vi "niRFUtil FTW Decimating FIR Filter (real wfm).vi"(0 "Waveform In":T1 {"y" min=0 max=127 format="%.2f"; "dx" format="%^.2e"; "x0" format="%^.2e"}, 5 "Filter":T1 {"y" min=0 max=127 format="%.2f"; "dx" format="%^.2e"; "x0" format="%^.2e"}, 7 "Decimating Factor":i32=1, 9 "Offset":i32) -> (4 "Waveform Out":T1 {"y" min=0 max=127 format="%.2f"; "dx" format="%^.2e"; "x0" format="%^.2e"})   [LabVIEW 2015, in "niRFUtil.lvlib"]
doc: "(c) Copyright 2006, National Instruments, Inc. This VI may not be duplicated, sold, or distributed without written consent from National Instruments."
uses:
  niRFUtil.lvlib
  Includes/niRFUtil INC Real Waveform.ctl
  Includes/niRFUtil INC Real Array.ctl
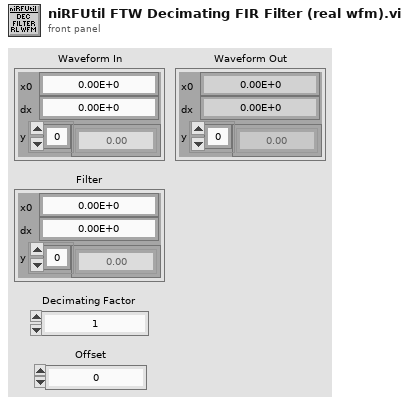
[diagram p1: front panel]
types:
  T1 = typedef "niRFUtil.lvlib/niRFUtil INC Real Waveform.ctl" = cluster{"x0":dbl, "dx":dbl, "y":T2}
  T2 = typedef "niRFUtil.lvlib/niRFUtil INC Real Array.ctl" = sgl[]
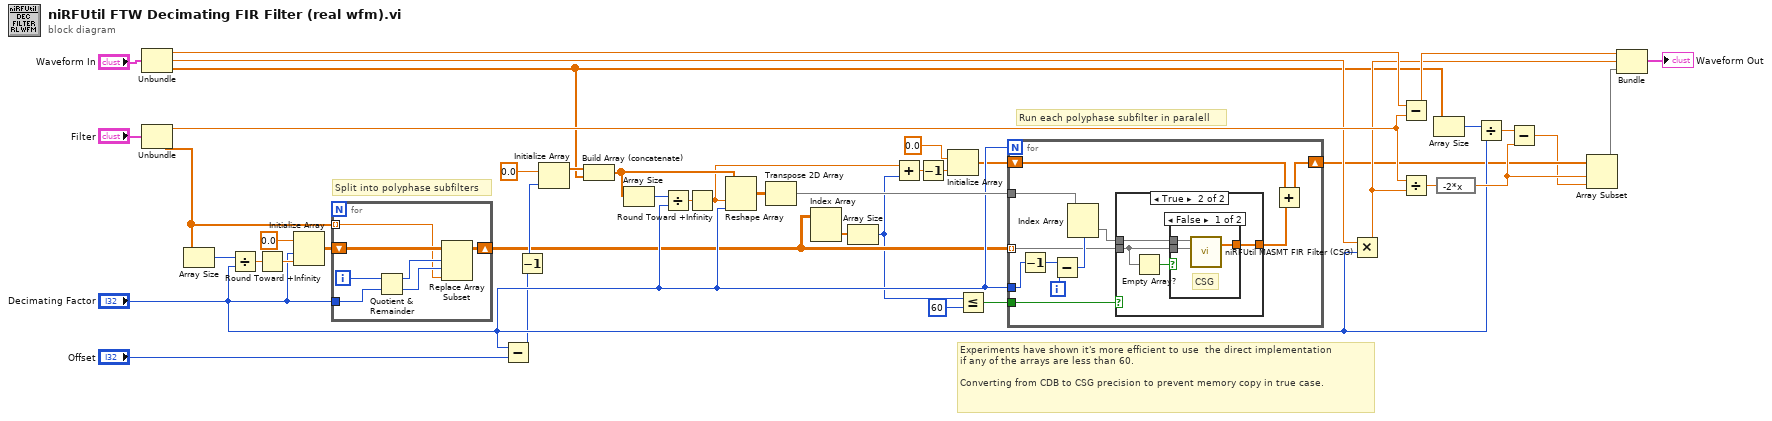
[diagram p0: block diagram]
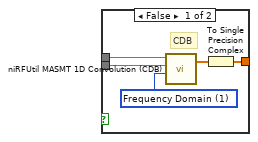
[diagram p2: hidden frame]
diagram:
  # "Experiments have shown it's more efficient to use  the direct implementation\nif any of the arrays are less than 60. \n\nConverting from CDB to CSG precision to prevent memory copy in true case."
  # "Run each polyphase subfilter in paralell"
  # "Split into polyphase subfilters"
  n1 = Unbundle("Waveform In") -> ("x0"=w33:dbl, "dx"=w27:dbl, "y"=w19:T2)
  n2 = Unbundle("Filter") -> ("x0"=w32:dbl, "y"=w38:T2)  [unwired: 1 out]
  n3 = Array Size(array=w38) -> (size(s)=w43:i32)
  n4 = Divide(x=w43, y="Decimating Factor") -> (x/y=w42:dbl)
  n5 = Round Toward +Infinity(x=w42) -> (ceil(x): smallest int >= x=w39:dbl)
  n6 = Initialize Array(sgl 0.0 ("element"), "Decimating Factor", w39) -> (w40:sgl[][])
  n7 = for {
    tunnel: w38 -> [w45] mode=indexing
    tunnel: "Decimating Factor" -> [w50]
    shift-right: [w44] -> w14
    shift-left: w40 -> [w48]
    i -> [w49]
    n8 = Quotient & Remainder(x=w49, y=w50) -> (x-y*floor(x/y)=w47:i32, floor(x/y)=w46:i32)
    n9 = Replace Array Subset(array=w48, new element=w45, index (row)=w47, index (col)=w46) -> (w44:sgl[][])
  }
  n10 = Subtract(x="Decimating Factor", y="Offset") -> (x-y=w16:i32)
  n11 = Decrement(x=w16) -> (x-1=w15:i32)
  n12 = Initialize Array(sgl 0.0 ("element"), w15) -> (w24:sgl[])
  n13 = Build Array (concatenate)(w24, w19) -> (w23:T2)
  n14 = Array Size(array=w23) -> (size(s)=w30:i32)
  n15 = Divide(x=w30, y="Decimating Factor") -> (x/y=w28:dbl)
  n16 = Round Toward +Infinity(x=w28) -> (ceil(x): smallest int >= x=w12:dbl)
  n17 = Reshape Array(w23, w12, "Decimating Factor") -> (w29:sgl[][])
  n18 = Transpose 2D Array(2D array=w29) -> (transposed array=w22:sgl[][])
  n19 = Index Array(array=w14) -> (element=w13:sgl[])  [unwired: 2 in]
  n20 = Array Size(array=w13) -> (size(s)=w2:i32)
  n21 = Add(x=w12, y=w2) -> (x+y=w11:dbl)
  n22 = Decrement(x=w11) -> (x-1=w8:dbl)
  n23 = Initialize Array(sgl 0.0, w8) -> (w10:sgl[])
  n24 = Less Or Equal?(x=w2, y=60) -> (x <= y?=w1:bool)
  n25 = for {
    N: "Decimating Factor" -> [_]
    tunnel: w14 -> [w54] mode=indexing
    tunnel: "Decimating Factor" -> [w61]
    tunnel: w22 -> [w58]
    shift-right: [w55] -> w7
    shift-left: w10 -> [w56]
    tunnel: w1 -> [w51]
    i -> [w60]
    n26 = Decrement(x=w61) -> (x-1=w59:i32)
    n27 = Subtract(x=w59, y=w60) -> (x-y=w57:i32)
    n28 = Index Array(array=w58, index (row)=w57) -> (element=w53:sgl[])  [unwired: 1 in]
    n29 = case shown="True" w51 {
      tunnel: [w62 w70] -> w52
      tunnel: w53 -> [w64 w69]
      tunnel: w54 -> [w65 w67]
      frame False {
        w66 = 1 items=["Direct", "Frequency Domain"] ("algorithm")
        # "CDB"
        n30 = call "niRFUtil MASMT 1D Convolution (CDB).vi"("algorithm"=w66, "Y"=w65, "X"=w64) -> ("X * Y"=w63:cdb[])  [unwired: 7 in, 1 out]
        n31 = To Single Precision Complex(1:w63) -> (0:w62:csg[])
      }
      frame True {
        n32 = Empty Array?(array=w67) -> (empty?=w68:bool)
        n33 = case shown="False" w68 {
          tunnel: [w73 _] -> w70
          tunnel: w69 -> [w72 _]
          tunnel: w67 -> [w71 _]
          frame False {
            # "CSG"
            n34 = call "niRFUtil MASMT FIR Filter (CSG).vi"("FIR Coefficients"=w71, "X"=w72) -> ("Filtered X"=w73:csg[])  [unwired: 8 in, 1 out]
          }
          frame True {
          }
        }
      }
    }
    n35 = Add(x=w56, y=w52) -> (x+y=w55:csg[])
  }
  n36 = Multiply(x=w27, y="Decimating Factor") -> (x*y=w26:dbl)
  n37 = Subtract(x=w33, y=w32) -> (x-y=w36:dbl)
  n38 = Divide(x=w32, y=w26) -> (x/y=w35:dbl)
  n39 = Array Size(array=w19) -> (size(s)=w21:i32)
  n40 = expression code="-2*x"(w35) -> (w31:dbl)
  n41 = Divide(x=w21, y="Decimating Factor") -> (x/y=w20:dbl)
  n42 = Subtract(x=w20, y=w31) -> (x-y=w4:dbl)
  n43 = Array Subset(array=w7, index=w31, length=w4) -> (w37:csg[])
  n44 = Bundle(w36, w26, w37) -> (→"Waveform Out":cluster{dbl, dbl, csg[]})  [unwired: 1 out]
